vi "Configure Source Function Type.vi"(8 "error in (no error)":errorcluster, 10 "Mode(0:Voltage)":u16(ring) items=["Voltage", "Current"], 11 "VISA resource name":refnum<visa-resource-name>) -> (0 "error out":errorcluster, 3 "VISA resource name out":refnum<visa-resource-name>)   [LabVIEW 2015, in "IT6000C.lvlib"]
doc: "This command is used to set the operating mode of the power supply.\n\n<b>mode</b>\n0:Voltage\n1:Current"
uses:
  <instrlib>/IT6000C/IT6000C.lvlib
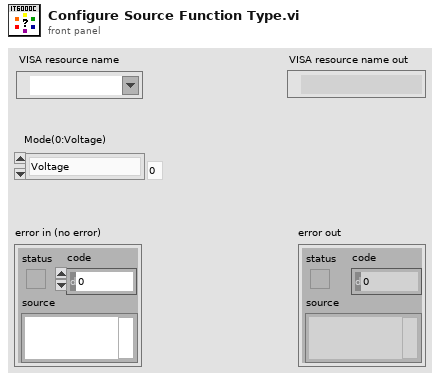
[diagram p1: front panel]
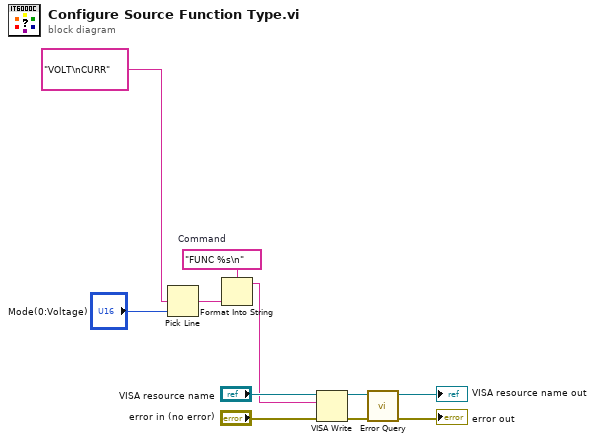
[diagram p0: block diagram]
diagram:
  w5 = "FUNC %s\n"  # Command
  n1 = Pick Line(multi-line string="VOLT\nCURR", line index="Mode(0:Voltage)") -> (output string=w1:string)  [unwired: 1 in]
  n2 = Format Into String(format string=w5, w1) -> (resulting string=w4:string)  [unwired: 2 in, 1 out]
  n3 = VISA Write(VISA resource name="VISA resource name", write buffer=w4, error in (no error)="error in (no error)") -> (VISA resource name out=w8:refnum<visa-resource-name>, error out=w9:errorcluster)  [unwired: 1 out]
  n4 = call <instrlib>:"Error Query.vi"("error in (no error)"=w9, "VISA resource name"=w8) -> ("error out"=→"error out":errorcluster, "VISA resource name out"=→"VISA resource name out":refnum<visa-resource-name>)  [unwired: 6 in, 2 out]
